vi "UpdateCfgIni.vi"(8 "error in":errorcluster, 10 "contentArray":string[](array[string]), 11 "iniCfgRefnumIn":refnum<file>) -> (0 "error out":errorcluster)   [LabVIEW 2010]
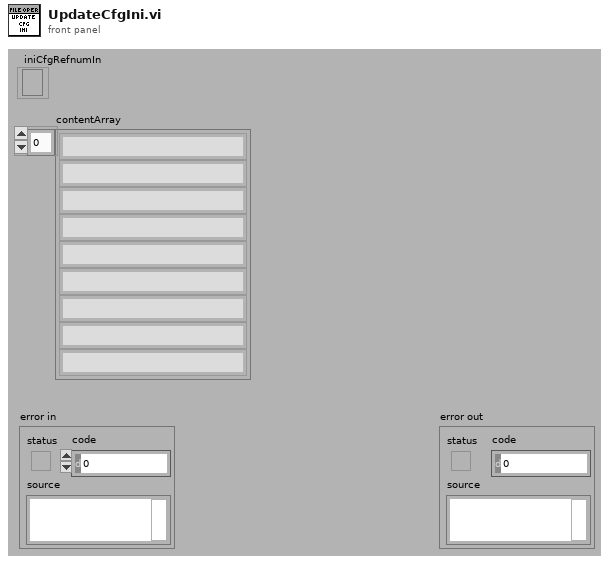
[diagram p1: front panel]
types:
  T1 = enum16{"open", "replace", "create", "open or create", "replace or create", "replace or create with confirmation"}
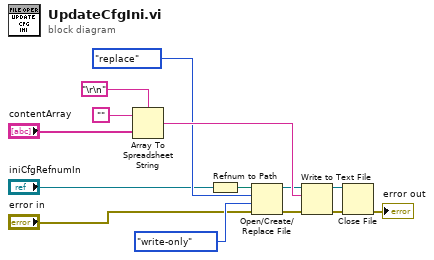
[diagram p0: block diagram]
diagram:
  n1 = Array To Spreadsheet String(delimiter (Tab)="\r\n", array="contentArray", 3:"") -> (spreadsheet string=w9:string)
  n2 = Refnum to Path(1:"iniCfgRefnumIn") -> (0:w5:path)
  n3 = Open/Create/Replace File(file path (use dialog)=w5, error in="error in", operation (0:open)=T1."replace", access (0:read/write)=enum16{"read/write", "read-only", "write-only"}."write-only") -> (refnum out=w8:refnum<file>, error out=w10:errorcluster)  [unwired: 2 in, 1 out]
  n4 = Write to Text File(file (use dialog)=w8, text=w9, error in=w10) -> (refnum out=w12:refnum<file>, error out=w13:errorcluster)  [unwired: 1 in, 1 out]
  n5 = Close File(refnum=w12, error in=w13) -> (error out=→"error out":errorcluster)  [unwired: 1 out]
